vi "Fade Out.vi"(7 "Stop Demo":refnum<user-event>, 8 "error in":errorcluster, 11 "Main Subpanel":refnum<vi>) -> (0 "error out":errorcluster)   [LabVIEW 2020]
uses:
  <vilib>/Utility/miscctls.llb/LVRectTypeDef.ctl
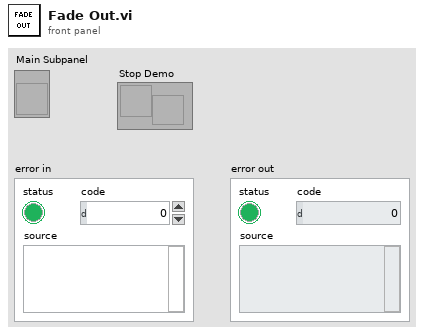
[diagram p1: front panel]
types:
  T1 = enum32{"Invalid", "Standard", "Closed", "Hidden", "Minimized", "Maximized"}
  T2 = typedef "LVRectTypeDef.ctl" = cluster{"Left":i16, "Top":i16, "Right":i16, "Bottom":i16}
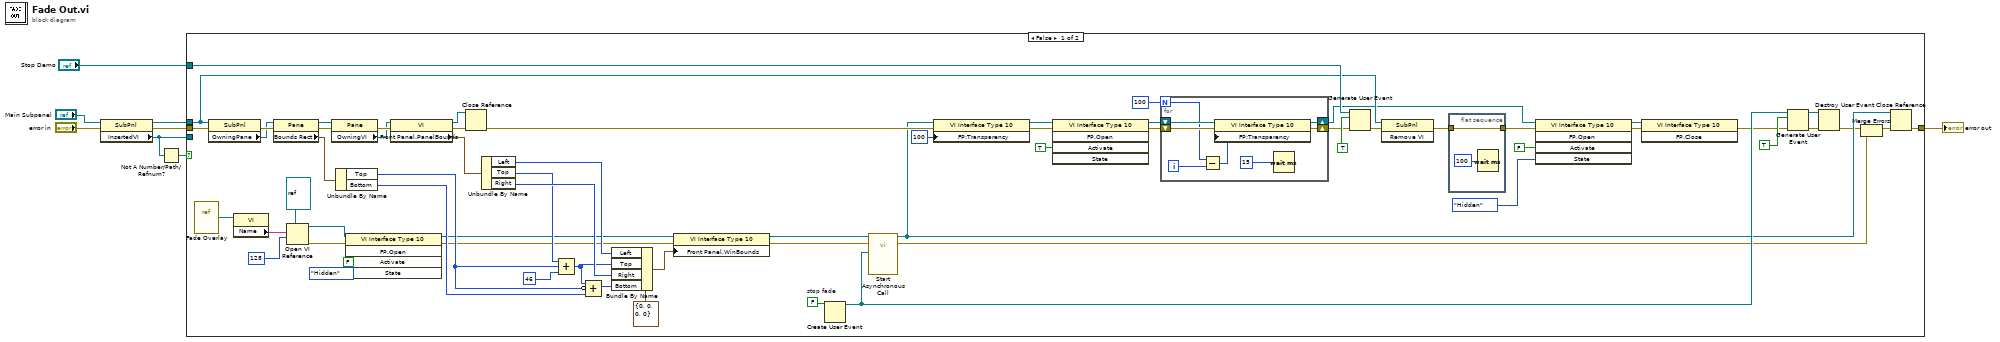
[diagram p0: block diagram]
diagram:
  n1 = property class="SubPnl"(reference="Main Subpanel", error in="error in") -> (reference out=w3:refnum<vi>, error out=w7:errorcluster, "InsertedVI"=w2:refnum<vi>)
  n2 = Not A Number/Path/Refnum?(number/path/refnum=w2) -> (NaN/Path/Refnum?=w4:bool)
  n3 = case shown="False" w4 {
    tunnel: w7 -> [w66 w83]
    tunnel: w3 -> [w65 _]
    tunnel: w2 -> [_ _]
    tunnel: [w46 w83] -> w6
    tunnel: "Stop Demo" -> [w71 _]
    frame False {
      w67 = FALSE  # stop fade
      n4 = vi-ref "Fade Overlay.vi"() -> (w56:refnum<vi>)
      n5 = property class="SubPnl"(reference=w65, error in=w66) -> (error out=w64:errorcluster, "OwningPane"=w63:refnum<vi>)  [unwired: 1 out]
      n6 = property class="VI"(reference=w56) -> ("Name"=w55:string)  [unwired: 1 in, 2 out]
      n7 = property class="Pane"(reference=w63, error in=w64) -> (reference out=w61:refnum<vi>, error out=w62:errorcluster, "Bounds Rect"=w37:T2)
      n8 = Open VI Reference(type specifier VI Refnum (for type only)=refnum<vi> refnum, vi path=w55, options=128) -> (vi reference=w13:refnum<vi>, error out=w14:errorcluster)  [unwired: 3 in]
      n9 = property class="Pane"(reference=w61, error in=w62) -> (error out=w60:errorcluster, "OwningVI"=w59:refnum<vi>)  [unwired: 1 out]
      n10 = Unbundle By Name(w37) -> ("Top"=w29:i16, "Bottom"=w30:i16)
      n11 = invoke class="VI Interface Type 10" method="FP.Open"(reference=w13, error in=w14, "Activate"=FALSE ("Activate?"), "State"=T1."Hidden") -> (reference out=w11:refnum<vi>, error out=w12:errorcluster)  [unwired: 1 in, 3 out]
      n12 = property class="VI"(reference=w59, error in=w60) -> (reference out=w57:refnum<vi>, error out=w58:errorcluster, "Front Panel.PanelBounds"=w36:T2)
      n13 = Close Reference(reference=w57, error in (no error)=w58) -> (error out=w52:errorcluster)
      n14 = Unbundle By Name(w36) -> ("Left"=w35:i16, "Top"=w33:i16, "Right"=w34:i16)
      n15 = Compound Arithmetic op=ADD(w33, w29, i16 46 ("value")) -> (w32:i16)
      n16 = Compound Arithmetic op=ADD(w32, invert w29, w30) -> (w31:i16)
      n17 = Bundle By Name(cluster=T2 {"Left"=0, "Top"=0, "Right"=0, "Bottom"=0} ("Front Panel Window:Panel Bounds"), "Left"=w35, "Top"=w32, "Right"=w34, "Bottom"=w31) -> (w38:T2)
      n18 = property class="VI Interface Type 10"(reference=w11, error in=w12, "Front Panel.WinBounds"=w38) -> (reference out=w9:refnum<vi>, error out=w10:errorcluster)
      n19 = Create User Event(user event datatype=w67) -> (user event=w49:refnum<user-event>)  [unwired: 1 in, 1 out]
      n20 = call-by-ref "Start Asynchronous Call"(reference=w9, error in=w10, "Stop Fade"=w49) -> (reference out=w43:refnum<vi>, error out=w44:errorcluster)  [unwired: 11 in]
      n21 = property class="VI Interface Type 10"(reference=w43, error in=w52, "FP:Transparency"=u8 100 ("Front Panel Window:Transparency")) -> (reference out=w41:refnum<vi>, error out=w50:errorcluster)
      n22 = invoke class="VI Interface Type 10" method="FP.Open"(reference=w41, error in=w50, "Activate"=TRUE ("Activate?")) -> (reference out=w40:refnum<vi>, error out=w42:errorcluster)  [unwired: 2 in, 3 out]
      n23 = for {
        N: 100 -> [w77]
        shift-right: [w79] -> w18
        shift-left: w40 -> [w80]
        shift-right: [w81] -> w26
        shift-left: w42 -> [w82]
        i -> [w75]
        n24 = Subtract(x=w77, y=w75) -> (x-y=w76:i32)
        n25 = property class="VI Interface Type 10"(reference=w80, error in=w82, "FP:Transparency"=w76) -> (reference out=w79:refnum<vi>, error out=w81:errorcluster)
        n26 = Wait (ms)(milliseconds to wait=u32 15) -> ()  [unwired: 1 out]
      }
      n27 = Generate User Event(user event=w71, event data cluster=TRUE ("event data"), error in=w26) -> (error out=w23:errorcluster)  [unwired: 1 in, 1 out]
      n28 = invoke class="SubPnl" method="Remove VI"(reference=w65, error in=w23) -> (error out=w22:errorcluster)  [unwired: 1 in, 2 out]
      n29 = flat-sequence {
        tunnel: [w74] -> w21
        tunnel: w22 -> [w74]
        frame #0 {
          n30 = Wait (ms)(milliseconds to wait=u32 100) -> ()  [unwired: 1 out]
        }
      }
      n31 = invoke class="VI Interface Type 10" method="FP.Open"(reference=w18, error in=w21, "Activate"=FALSE ("Activate?"), "State"=T1."Hidden") -> (reference out=w17:refnum<vi>, error out=w19:errorcluster)  [unwired: 1 in, 3 out]
      n32 = invoke class="VI Interface Type 10" method="FP.Close"(reference=w17, error in=w19) -> (error out=w27:errorcluster)  [unwired: 1 in, 2 out]
      n33 = Generate User Event(user event=w49, event data cluster=TRUE ("event data"), error in=w27) -> (user event out=w24:refnum<user-event>, error out=w47:errorcluster)  [unwired: 1 in]
      n34 = Destroy User Event(user event=w24, error in=w47) -> (error out=w25:errorcluster)
      n35 = Merge Errors(w25, w44) -> (w45:errorcluster)
      n36 = Close Reference(reference=w43, error in (no error)=w45) -> (error out=w46:errorcluster)
    }
    frame True {
    }
  }
  "error out" <- w6
